vi "editConfiguration.vi"(10 "ILCAppConfig":T1={"ILCConfig"={"Input Channels"=enum."Channel 0", "Scan Rate (Hz) "=enum."50", "ADC PGA Gain"=0}, "RS232Config"={"VISA resource name"="", "Baud Rate"=9600, "Data Bits"=8, "Parity"=enum."None", "Stop Bits"=10, "Flow Control"=0, "Timeout (ms)"=10000}, "Application Timing"={"Loop Period (ms)"=100}} {"Application Timing"."Loop Period (ms)" min=1 max=5000; "RS232Config"."Stop Bits" items=["1.0"=10, "1.5"=15, "2.0"=20]; "RS232Config"."Flow Control" items=["None", "XON/XOFF", "RTS/CTS", "XON/XOFF & RTS/CTS", "DTR/DSR", "XON/XOFF & DTR/DSR"]; "RS232Config"."Data Bits" min=5 max=8 step=1; "ILCConfig"."ADC PGA Gain" max=7}) -> (1 "canceledIsTrue":bool, 2 "ILCAppConfig 2":T1={"ILCConfig"={"Input Channels"=enum."Channel 0", "Scan Rate (Hz) "=enum."50", "ADC PGA Gain"=0}, "RS232Config"={"VISA resource name"="", "Baud Rate"=9600, "Data Bits"=8, "Parity"=enum."None", "Stop Bits"=10, "Flow Control"=0, "Timeout (ms)"=10000}, "Application Timing"={"Loop Period (ms)"=1}} {"Application Timing"."Loop Period (ms)" min=1 max=5000; "RS232Config"."Stop Bits" items=["1.0"=10, "1.5"=15, "2.0"=20]; "RS232Config"."Flow Control" items=["None", "XON/XOFF", "RTS/CTS", "XON/XOFF & RTS/CTS", "DTR/DSR", "XON/XOFF & DTR/DSR"]; "RS232Config"."Data Bits" min=5 max=8 step=1; "ILCConfig"."ADC PGA Gain" max=7})   [LabVIEW 2012]
uses:
  State/ILCAppConfig.ctl
  Configuration/ILCConfig.ctl
  Configuration/InputChannels.ctl
  Configuration/ScanRate_Hz_MultichannelOptions.ctl
  Configuration/RS232Config.ctl
  Model/Model/ApplicationTiming.ctl
panel:
  in  "CancelIsTrue":bool
  in  "OKIsTrue":bool
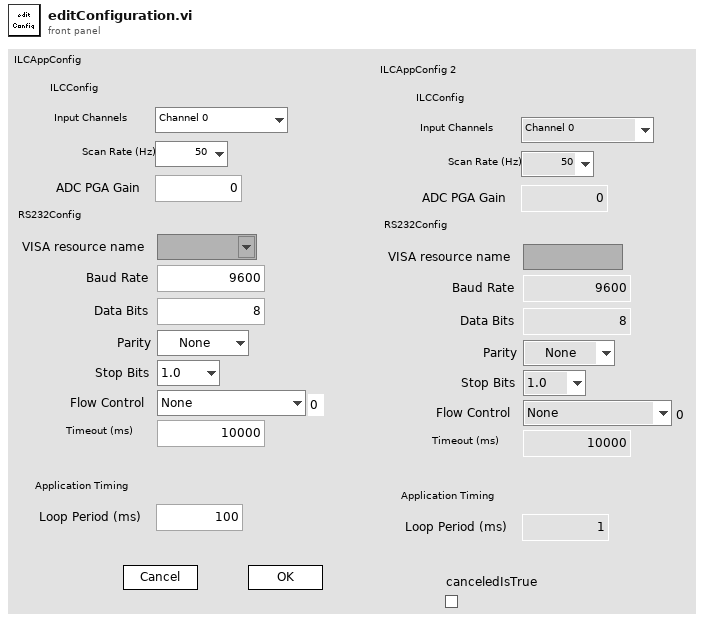
[diagram p1: front panel]
types:
  T1 = typedef "ILCAppConfig.ctl" = cluster{"ILCConfig":T2, "RS232Config":T5, "Application Timing":T6}
  T2 = typedef "ILCConfig.ctl" = cluster{"Input Channels":T3, "Scan Rate (Hz) ":T4, "ADC PGA Gain":u8}
  T3 = typedef "InputChannels.ctl" = enum16{"Channel 0", "3 Channels", "5 Channels"}
  T4 = typedef "ScanRate_Hz_MultichannelOptions.ctl" = enum16{"50", "60", "100", "120", "200", "240", "300", "400", "480", "600", "1200", "2400", "4800"}
  T5 = typedef "RS232Config.ctl" = cluster{"VISA resource name":refnum<visa-resource-name>, "Baud Rate":u32, "Data Bits":u16, "Parity":enum16{"None", "Odd", "Even", "Mark", "Space"}, "Stop Bits":u16, "Flow Control":u16, "Timeout (ms)":u32}
  T6 = typedef "ApplicationTiming.ctl" = cluster{"Loop Period (ms)":u16}
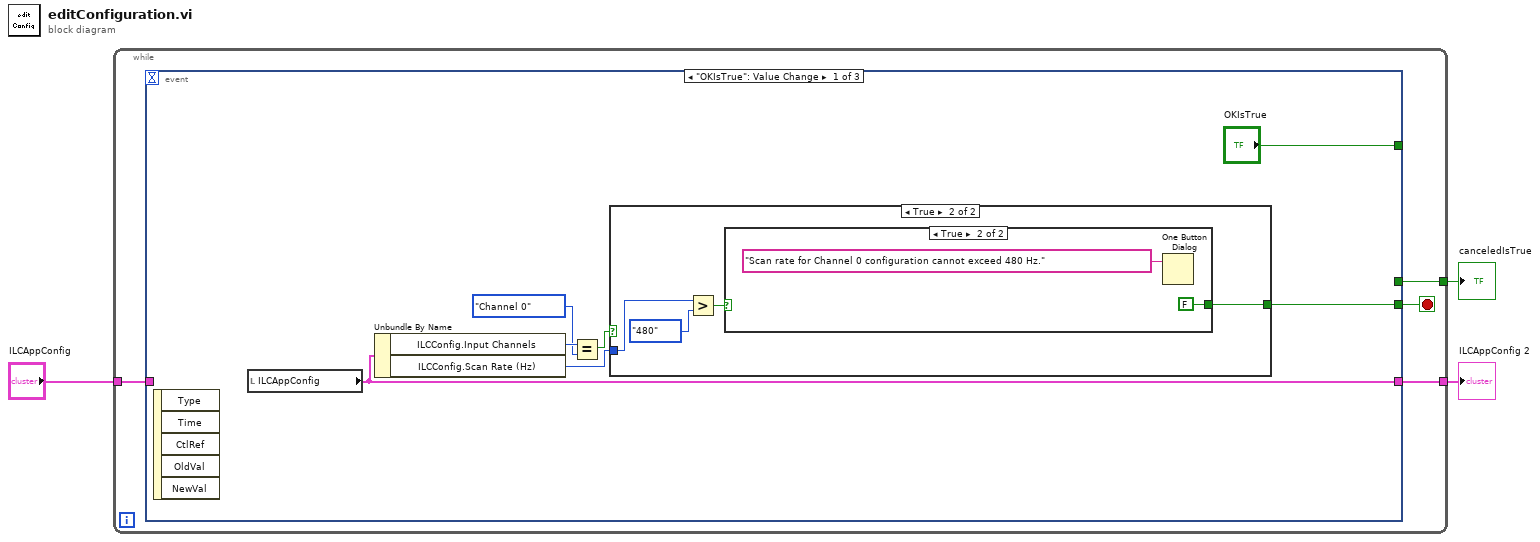
[diagram p0: block diagram]
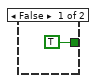
[diagram p2: hidden frame]
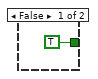
[diagram p3: hidden frame]
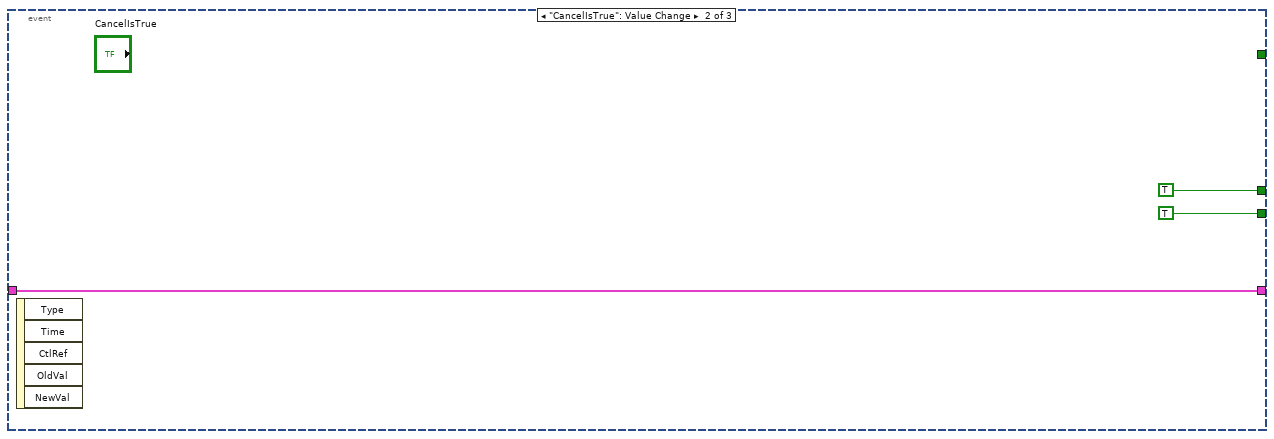
[diagram p4: hidden frame]
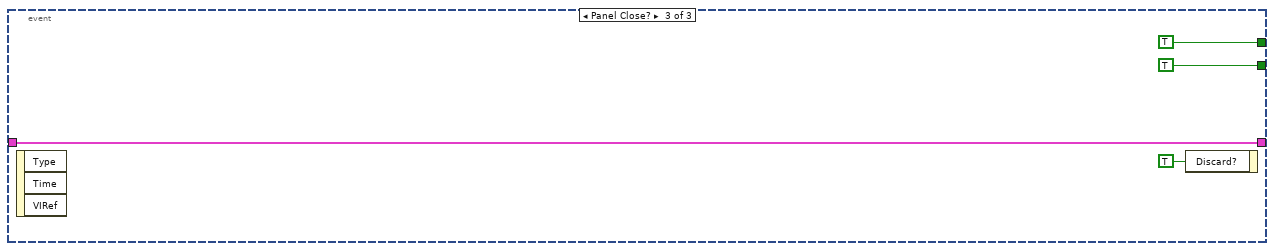
[diagram p5: hidden frame]
diagram:
  n1 = while {
    tunnel: [w7] -> w3
    tunnel: [w6] -> w2
    tunnel: "ILCAppConfig" -> [w5]
    stop <- w4 stop-if-true
    n2 = event shown="[0] \"OKIsTrue\": Value Change" {
      selector: _ -> [_ _ _]
      dyn-events: _ -> [_ _ _]
      timeout: _ -> [_ _ _]
      tunnel: ["OKIsTrue" _ _] -> _
      tunnel: [_ TRUE ("Discard?") TRUE ("Discard?")] -> w7
      tunnel: [w13 w24 w27] -> w6
      tunnel: w5 -> [_ w24 w27]
      tunnel: [w8 TRUE TRUE] -> w4
      event "OKIsTrue": Value Change {
        n3 = event-data() -> ()  [unwired: 1 in, 5 out]
        n4 = local read "ILCAppConfig"() -> (w13:T1)
        n5 = Unbundle By Name(w13) -> ("ILCConfig.Input Channels"=w12:T3, "ILCConfig.Scan Rate (Hz)"=w9:T4)
        n6 = Equal?(x=w12, y=InputChannels."Channel 0") -> (x = y?=w10:bool)
        n7 = case shown="True" w10 {
          tunnel: w9 -> [_ w19]
          tunnel: [TRUE w16] -> w8
          frame False {
          }
          frame True {
            n8 = Greater?(x=w19, y=ScanRate_Hz_MultichannelOptions."480") -> (0:w17:bool)
            n9 = case shown="True" w17 {
              tunnel: [TRUE FALSE] -> w16
              frame False {
              }
              frame True {
                n10 = One Button Dialog(message="Scan rate for Channel 0 configuration cannot exceed 480 Hz.") -> ()  [unwired: 1 in, 1 out]
              }
            }
          }
        }
      }
      event "CancelIsTrue": Value Change {
        n11 = event-data() -> ()  [unwired: 1 in, 5 out]
      }
      event Panel Close? {
        n12 = event-data() -> ()  [unwired: 1 in, 3 out]
        n13 = event-data("Discard?"=TRUE) -> ()  [unwired: 1 in, 1 out]
      }
    }
  }
  "canceledIsTrue" <- w3
  "ILCAppConfig 2" <- w2
